vi "GRIMMstatusGFV.vi"(8 "error in (no error)":errorcluster, 10 "Variant in":variant, 11 "GrimmStatusEnum":T1=enum."Insert Status Data") -> (0 "error out":errorcluster, 3 "Variant out":variant)   [LabVIEW 2013]
doc: "Use this template to build a VI to use as a subVI."
uses:
  GRIMMstatusEnum.ctl
  <vilib>/Utility/miscctls.llb/LVDateTimeRec.ctl
  GRIMMStatusCluster.ctl
  GRIMMErrorMessage.ctl
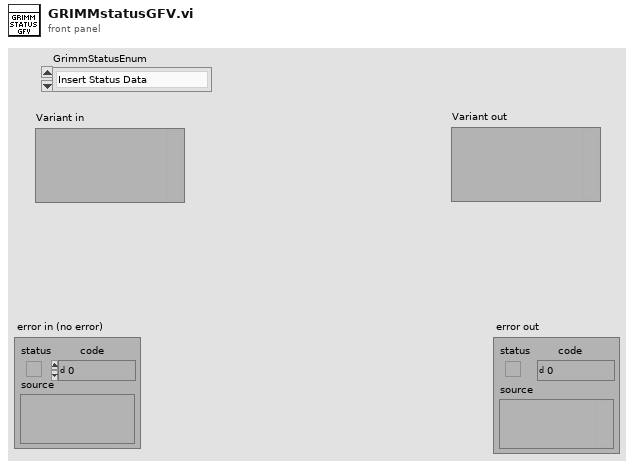
[diagram p1: front panel]
types:
  T1 = typedef "GRIMMstatusEnum.ctl" = enum16{"Get Pump Current", "Get Power Supply Type", "Get Battery Power", "Get Error message", "Get Instrument DateTime", "Insert Status Data", "Init"}
  T2 = enum16{"220 Volt Network Grid", "Battery Powered"}
  T3 = typedef "LVDateTimeRec.ctl" = cluster{"fractional second":dbl, "second":i32, "minute":i32, "hour":i32, "day of month":i32, "month":i32, "year":i32, "day of week":i32, "day of year":i32, "DST":i32}
  T4 = typedef "GRIMMStatusCluster.ctl" = cluster{"Time Stamp":timestamp, "Location Number":i32, "Gravimetric Factor":i32, "Battery Power %":i32, "Pump Current %":i32, "Power Supply":enum16{"220 Volt Network Grid", "Battery Powered"}, "External Sensor Input":i32[], "Error Messages":T5}
  T5 = typedef "GRIMMErrorMessage.ctl" = u16
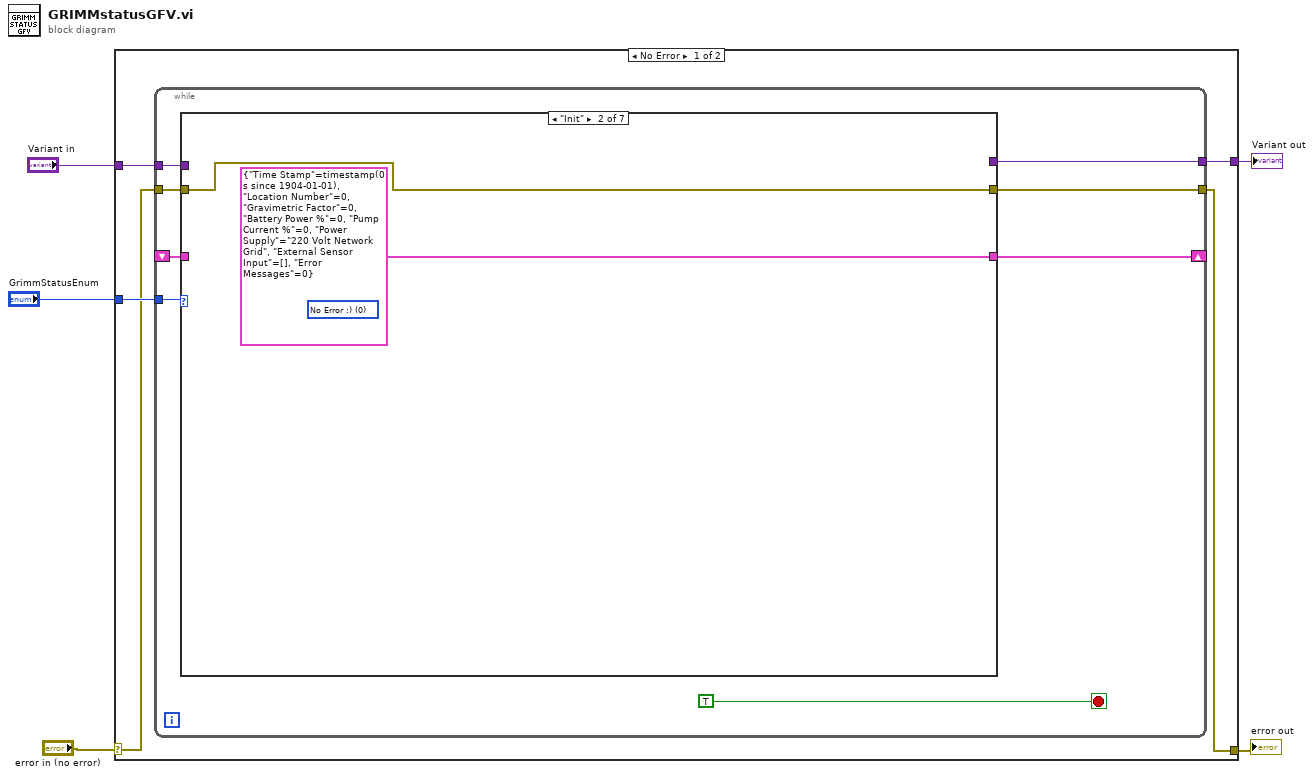
[diagram p0: block diagram]
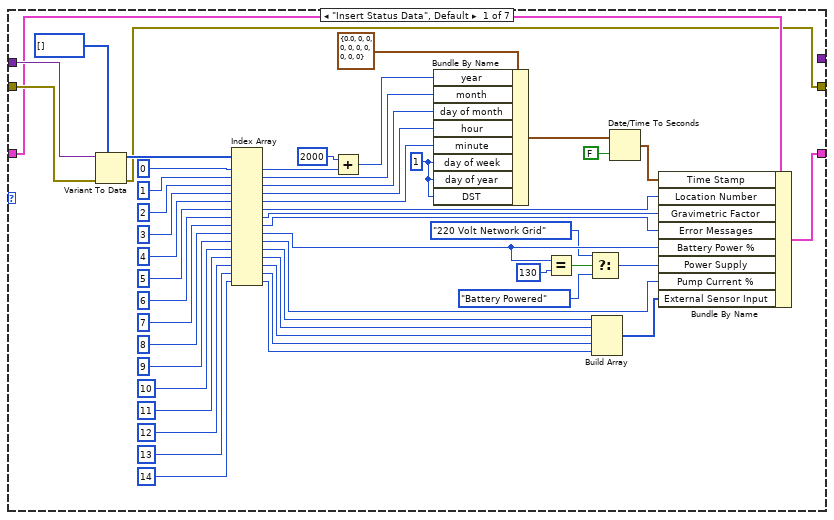
[diagram p2: hidden frame]
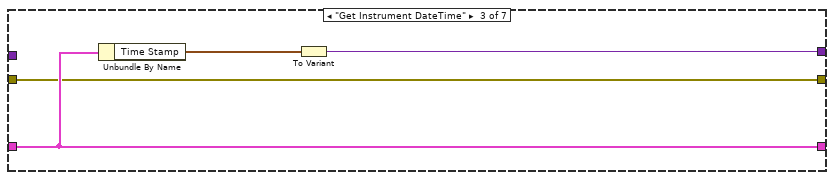
[diagram p3: hidden frame]
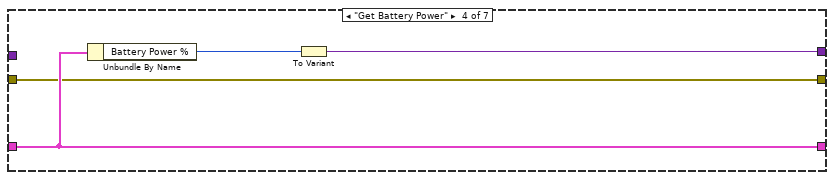
[diagram p4: hidden frame]
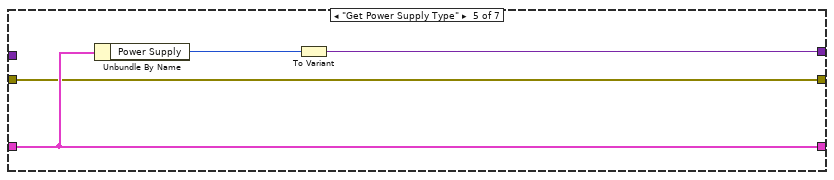
[diagram p5: hidden frame]
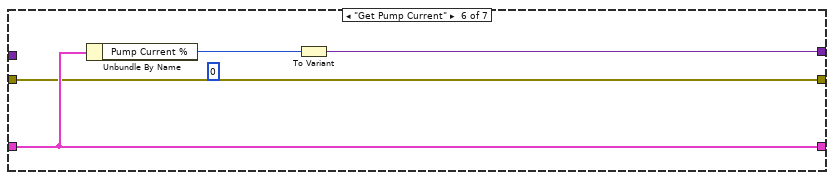
[diagram p6: hidden frame]
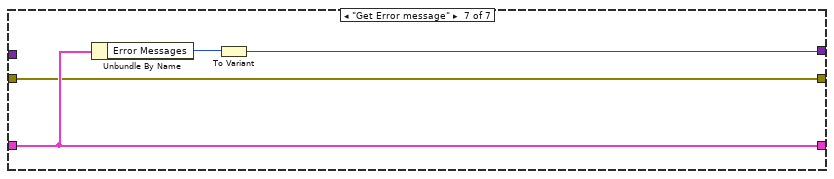
[diagram p7: hidden frame]
diagram:
  n1 = case shown="No Error" "error in (no error)" {
    selector: "error in (no error)" -> [w8 w91]
    tunnel: [w6 w91] -> w4
    tunnel: "GrimmStatusEnum" -> [w10 _]
    tunnel: "Variant in" -> [w9 _]
    tunnel: [w7 _] -> w1
    frame No Error {
      n2 = while {
        tunnel: w10 -> [w17]
        shift-right: [w16] -> _
        shift-left: _ -> [w15]
        tunnel: w9 -> [w14]
        tunnel: w8 -> [w13]
        tunnel: [w12] -> w7
        tunnel: [w11] -> w6
        stop <- TRUE stop-if-true
        n3 = case shown="\"Init\"" w17 {
          tunnel: [w48 T4 {"Time Stamp"=timestamp(0 s since 1904-01-01), "Location Number"=0, "Gravimetric Factor"=0, "Battery Power %"=0, "Pump Current %"=0, "Power Supply"=enum."220 Volt Network Grid", "External Sensor Input"=[], "Error Messages"=0} w74 w78 w82 w86 w90] -> w16
          tunnel: w15 -> [w66 _ w74 w78 w82 w86 w90]
          tunnel: w14 -> [w68 _ _ _ _ _ _]
          tunnel: w13 -> [w67 w69 w73 w77 w81 w85 w89]
          tunnel: [_ _ w71 w75 w79 w83 w87] -> w12
          tunnel: [w19 w69 w73 w77 w81 w85 w89] -> w11
          frame "Insert Status Data", Default {
            w46 = 1 ("DST")
            n4 = Variant To Data(error in=w67, type=i32[] [] ("Output Number of Particles per 100 CC"), Variant=w68) -> (data=w63:i32[], error out=w19:errorcluster)
            n5 = Index Array(array=w63, index #1=0 ("index"), index #2=1 ("index"), index #3=2 ("index"), index #4=3 ("index"), index #5=4 ("index"), index #6=5 ("index"), index #7=6 ("index"), index #8=7 ("index"), index #9=8 ("index"), index #10=9 ("index"), index #11=10 ("index"), index #12=11 ("index"), index #13=12 ("index"), index #14=13 ("index"), index #15=14 ("index")) -> (element #1=w57:i32, element #2=w54:i32, element #3=w53:i32, element #4=w52:i32, element #5=w51:i32, element #6=w44:i32, element #7=w42:i32, element #8=w40:i32, element #9=w37:i32, element #10=w31:i32, element #11=w25:i32, element #12=w24:i32, element #13=w23:i32, element #14=w22:i32, element #15=w21:i32)
            n6 = Add(x=2000, y=w57) -> (x+y=w55:i32)
            n7 = Bundle By Name(cluster=T3 {"fractional second"=0.0, "second"=0, "minute"=0, "hour"=0, "day of month"=0, "month"=0, "year"=0, "day of week"=0, "day of year"=0, "DST"=0} ("date time rec"), "year"=w55, "month"=w54, "day of month"=w53, "hour"=w52, "minute"=w51, "day of week"=w46, "day of year"=w46, "DST"=w46) -> (w50:T3)
            n8 = Equal?(x=w37, y=130) -> (x = y?=w38:bool)
            n9 = Select(t=T2."220 Volt Network Grid" ("Power Supply"), s=w38, f=T2."Battery Powered" ("Power Supply")) -> (s? t:f=w33:T2)
            n10 = Build Array(w25, w24, w23, w22, w21) -> (w20:i32[])
            n11 = Date/Time To Seconds(1:FALSE ("is UTC (F)"), 2:w50) -> (0:w49:timestamp)
            n12 = Bundle By Name(cluster=w66, "Time Stamp"=w49, "Location Number"=w44, "Gravimetric Factor"=w42, "Error Messages"=w40, "Battery Power %"=w37, "Power Supply"=w33, "Pump Current %"=w31, "External Sensor Input"=w20) -> (w48:T4)
          }
          frame "Init" {
            (unwired) T5 0 items=["New SELF-TEST: Fault Self-Test"=128, "No Memory Card"=64, "Check Nozzle: Whirls > 5%"=32, "No Operation: Battery Capacity = 0%"=16, "Please Recharge: Battery Capacity < 10%"=8, "Pump Current too High - Motor Current Imot > 100%"=4, "Flow-Error: Volume flow control out of control range"=3, "Check Filter Imot < 20% "=2, "Check Filter Imot > 60%"=1, "No Error :)"=0] ("Error Messages")
          }
          frame "Get Instrument DateTime" {
            n13 = Unbundle By Name(w74) -> ("Time Stamp"=w72:timestamp)
            n14 = To Variant(anything=w72) -> (Variant=w71:variant)
          }
          frame "Get Battery Power" {
            n15 = Unbundle By Name(w78) -> ("Battery Power %"=w76:i32)
            n16 = To Variant(anything=w76) -> (Variant=w75:variant)
          }
          frame "Get Power Supply Type" {
            n17 = Unbundle By Name(w82) -> ("Power Supply"=w80:T2)
            n18 = To Variant(anything=w80) -> (Variant=w79:variant)
          }
          frame "Get Pump Current" {
            (unwired) 0 ("Pump Current %")
            n19 = Unbundle By Name(w86) -> ("Pump Current %"=w84:i32)
            n20 = To Variant(anything=w84) -> (Variant=w83:variant)
          }
          frame "Get Error message" {
            n21 = Unbundle By Name(w90) -> ("Error Messages"=w88:T5)
            n22 = To Variant(anything=w88) -> (Variant=w87:variant)
          }
        }
      }
    }
    frame Error {
    }
  }
  "error out" <- w4
  "Variant out" <- w1
